vi "Read Command Core.vi"(8 "error in (no error)":errorcluster, 9 "timeout ms (5000)":i32=5000, 10 "Data":string, 11 "Websocket Client Handler in":refnum<class "Websocket Client Handler.lvclass">) -> (0 "error out":errorcluster, 3 "Websocket Client Handler out":refnum<class "Websocket Client Handler.lvclass">)   [LabVIEW 2016, in "Stream Mediator.lvlib" / "Websocket Client Handler.lvclass"]
doc: "--\nCopyright © 2017 Composed SystemsI All rights reserved.\n\nAuthor: Jon McBee <jon.mcbee@composed.io>\n\nThis library is provided \"AS IS\" ,WITHOUT WARRANTIES OR\nCONDITIONS OF ANY KIND, either express or implied.\n\nComposed Systems -- composed.io\n\nStream 0.0.1.1\nJon McBee - Composed Systems\nCopyright (c) 2017, Composed Systems"
uses:
  <userlib>/Composed Systems/Stream/Mediator/Classes/Websocket Client Handler Actor/Websocket Client Handler/Websocket Client Handler.lvclass
  <userlib>/Composed Systems/Stream/Mediator/Classes/Websocket Client Handler Actor/Websocket Client Handler/Websocket Client Handler.lvclass/Websocket Client Handler.ctl
  <vilib>/MediaMongrels Ltd/WebSockets/WebSockets/WebSockets.lvlib
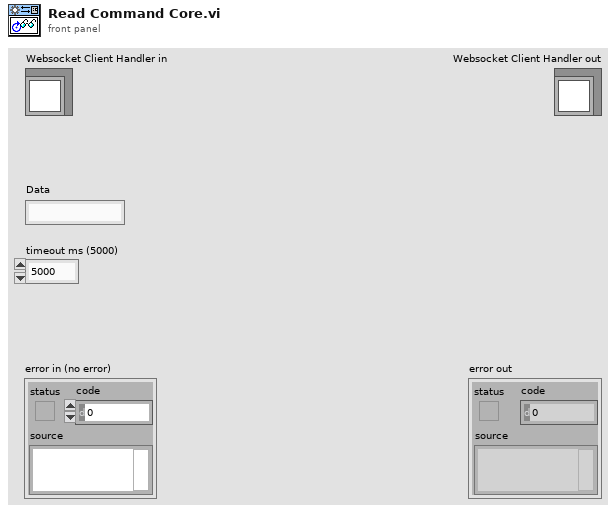
[diagram p1: front panel]
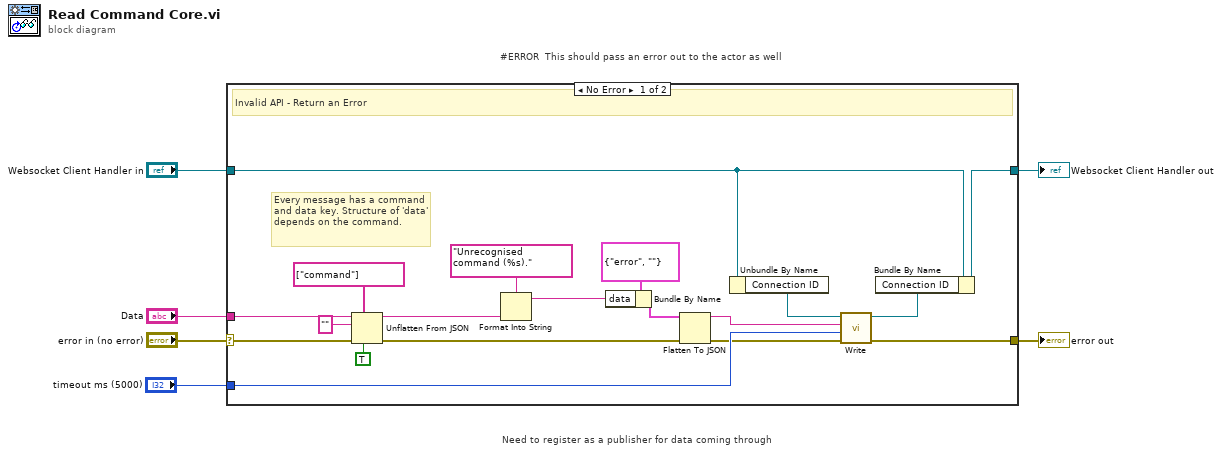
[diagram p0: block diagram]
diagram:
  # "Need to register as a publisher for data coming through"
  # "#ERROR  This should pass an error out to the actor as well"
  n1 = case shown="No Error" "error in (no error)" {
    selector: "error in (no error)" -> [w21 w27]
    tunnel: [w25 w27] -> w5
    tunnel: [w23 w26] -> w3
    tunnel: "Websocket Client Handler in" -> [w24 w26]
    tunnel: "Data" -> [w20 _]
    tunnel: "timeout ms (5000)" -> [w22 _]
    frame No Error {
      # "Every message has a command and data key. Structure of 'data' depends on the command."
      # "Invalid API - Return an Error"
      n2 = Unflatten From JSON(path=string[] ["command"], JSON string=w20, type and defaults="", default null elements? (F)=TRUE, error in (no error)=w21) -> (value=w7:string, error out=w8:errorcluster)  [unwired: 2 in]
      n3 = Format Into String(format string="Unrecognised command (%s).", w7) -> (resulting string=w16:string)  [unwired: 2 in, 1 out]
      n4 = Bundle By Name(cluster=cluster{"command":string, "data":string} {"command"="error", "data"=""}, "data"=w16) -> (w18:cluster{"command":string, "data":string})
      n5 = Flatten To JSON(anything=w18, error in (no error)=w8) -> (JSON string=w14:string, 11:w15:errorcluster)  [unwired: 1 in]
      n6 = Unbundle By Name(w24) -> ("Connection ID"=w13:refnum<k5>)
      n7 = call <vilib>:"Write.vi"("error in (no error)"=w15, "timeout ms (5000)"=w22, "Data"=w14, "WebSocket Connection in"=w13) -> ("error out"=w25:errorcluster, "WebSocket Connection out"=w12:refnum<k5>)  [unwired: 6 in]
      n8 = Bundle By Name(cluster=w24, "Connection ID"=w12) -> (w23:refnum<class "Websocket Client Handler.lvclass">)
    }
    frame Error {
    }
  }
  "error out" <- w5
  "Websocket Client Handler out" <- w3
